vi "Time.vi"(8 "error in (no error)":errorcluster, 10 "Control In":T1, 11 "Dispense Offset in":refnum<class "Dispense Offset.lvclass">) -> (0 "error out":errorcluster, 1 "Timing Data":i32[](array[numeric]), 2 "Control Out":T1, 3 "Dispense Offset out":refnum<class "Dispense Offset.lvclass">)   [LabVIEW 2019, in "Dispense Offset.lvclass"]
uses:
  Dispense Offset.lvclass
  Controller/Motion/A3200/A3200.lvclass
  Controller/Controllers.ctl
  Controller/Controller.lvclass
  Controller/I-O/I-O.lvclass
  Controller/Dispenser/Dispenser.lvclass
  C:/Program Files (x86)/Aerotech/A3200/LabVIEW/2010/Bin/Aerotech.A3200.dll
  Program Files (x86)/Aerotech/A3200/LabVIEW/2010/Bin/Aerotech.A3200.dll
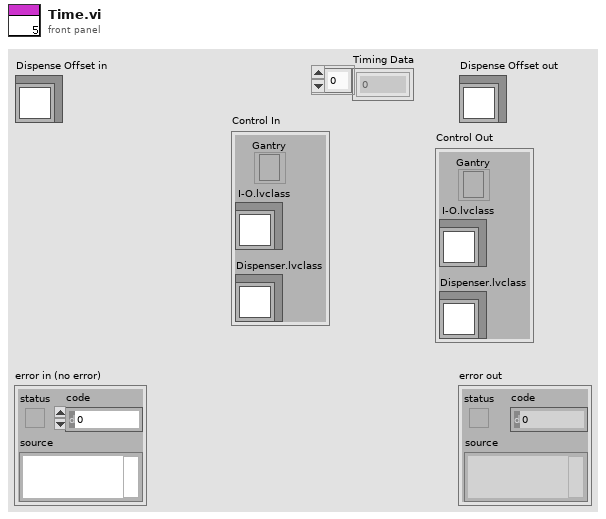
[diagram p1: front panel]
types:
  T1 = typedef "Controller.lvclass/Controllers.ctl" = cluster{"I-O.lvclass":refnum<class "I-O.lvclass">, "Dispenser.lvclass":refnum<class "Dispenser.lvclass">, "Gantry":refnum<k24>}
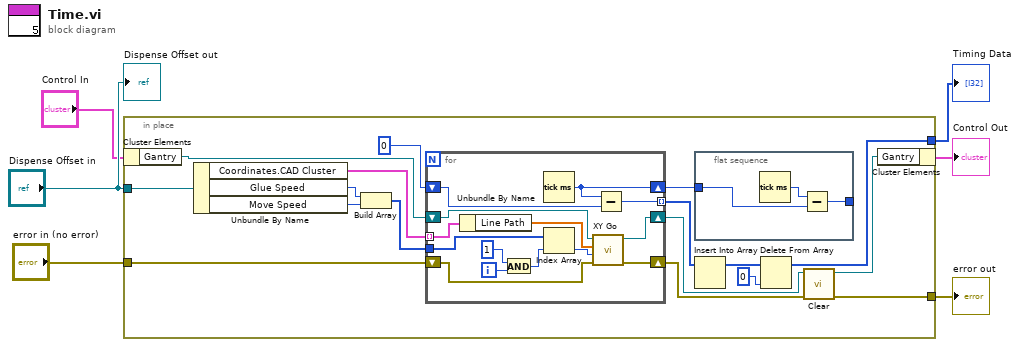
[diagram p0: block diagram]
diagram:
  n1 = in-place {
    in-place-border: "Dispense Offset in" -> [w23]
    in-place-border: "error in (no error)" -> [w16]
    in-place-border: [w12] -> w3
    in-place-border: [w7] -> w2
    n2 = in-place-cluster #1("Control In") -> ("Gantry"=w19:refnum<k24>)
    n3 = Unbundle By Name(w23) -> ("Coordinates.CAD Cluster"=w18:cluster{"Dispense?":bool, "Line Path":dbl[]}[], "Glue Speed"=w22:i32, "Move Speed"=w21:i32)
    n4 = Build Array(w22, w21) -> (w17:i32[])
    n5 = for {
      shift-right: [w35] -> w11
      shift-left: u32 0 ("millisecond timer value") -> [w38]
      tunnel: [w37] -> w8 mode=indexing
      tunnel: w17 -> [w33]
      shift-right: [w31] -> w15
      shift-left: w19 -> [w32]
      shift-right: [w29] -> w14
      shift-left: w16 -> [w30]
      tunnel: w18 -> [w28] mode=indexing
      i -> [w39]
      n6 = Unbundle By Name(w28) -> ("Line Path"=w27:dbl[])
      n7 = And(x=1, y=w39) -> (x .and. y?=w36:i32)
      n8 = Tick Count (ms)() -> (millisecond timer value=w35:u32)
      n9 = Index Array(array=w33, index=w36) -> (element=w34:i32)
      n10 = call "XY Go.vi"("error in (no error)"=w30, "Speed"=w34, "XY"=w27, "Gantry In"=w32) -> ("error out"=w29:errorcluster, "Gantry Out"=w31:refnum<k24>)  [unwired: 6 in]
      n11 = Subtract(x=w35, y=w38) -> (x-y=w37:u32)
    }
    n12 = flat-sequence {
      tunnel: [w25] -> _
      tunnel: w11 -> [w24]
      frame #0 {
        n13 = Tick Count (ms)() -> (millisecond timer value=w26:u32)
        n14 = Subtract(x=w26, y=w24) -> (x-y=w25:u32)
      }
    }
    n15 = Insert Into Array(array=w8) -> (w9:u32[])  [unwired: 2 in]
    n16 = Delete From Array(array=w9, index=0) -> (array with subset deleted=w7:u32[])  [unwired: 1 in, 1 out]
    n17 = call "Clear.vi"("error in (no error)"=w14, "Gantry In"=w15) -> ("error out"=w12:errorcluster, "Gantry Out"=w13:refnum<k24>)  [unwired: 8 in]
    n18 = in-place-cluster #1("Gantry"=w13) -> (→"Control Out":T1)
  }
  "error out" <- w3
  "Timing Data" <- w2
  "Dispense Offset out" <- "Dispense Offset in"
